vi "Print PDFCreator.vi"(0 "report in":refnum<class "NI_report.lvclass">, 2 "Printer name":string="PDFCreator", 5 "Save Directory":path, 7 "Save Filename":string="TEST", 11 "error in (no error)":errorcluster) -> (4 "report out":refnum<class "NI_report.lvclass">, 8 "File path":path, 15 "error out":errorcluster)   [LabVIEW 2010]
doc: "Jean-Marc Simard \nJanuary 6, 2010"
uses:
  <vilib>/Utility/NIReport.llb/NI_report.lvclass
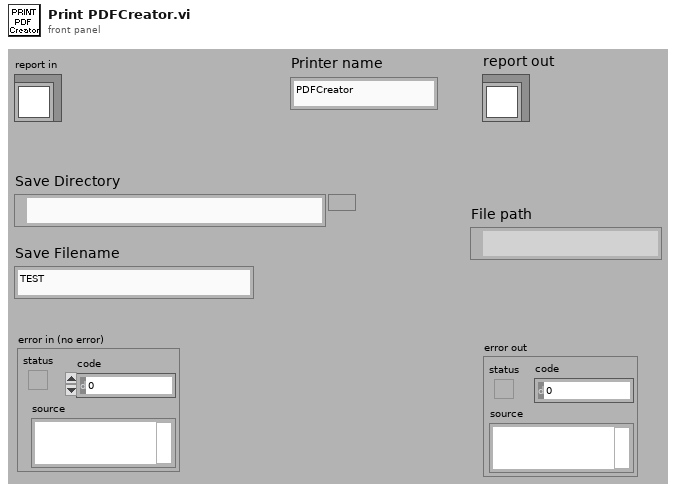
[diagram p1: front panel]
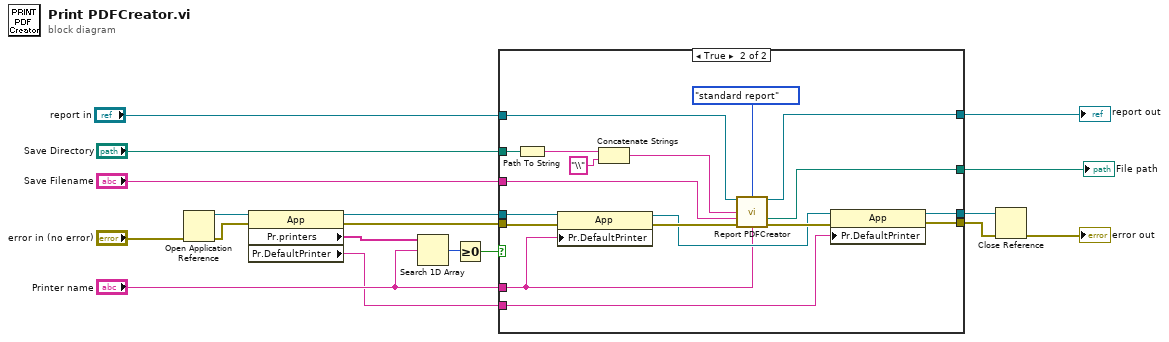
[diagram p0: block diagram]
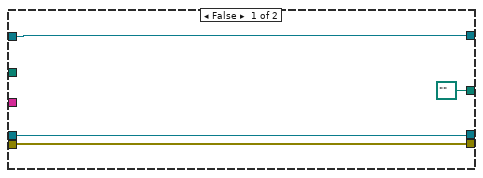
[diagram p2: hidden frame]
diagram:
  n1 = Open Application Reference(8:"error in (no error)") -> (0:w13:errorcluster, 3:w12:refnum<vi>)  [unwired: 3 out]
  n2 = property class="App"(reference=w12, error in=w13) -> (reference out=w8:refnum<vi>, error out=w7:errorcluster, "Pr.printers"=w11:string[], "Pr.DefaultPrinter"=w6:string)
  n3 = Search 1D Array(1D array=w11, element="Printer name") -> (index of element=w10:i32)  [unwired: 1 out]
  n4 = Greater Or Equal To 0?(x=w10) -> (x >= 0?=w9:bool)
  n5 = case shown="True" w9 {
    tunnel: w8 -> [w22 w40]
    tunnel: w7 -> [w21 w39]
    tunnel: "Printer name" -> [_ w23]
    tunnel: w6 -> [_ w25]
    tunnel: "Save Filename" -> [_ w35]
    tunnel: "Save Directory" -> [_ w34]
    tunnel: [w22 w33] -> w5
    tunnel: [w21 w32] -> w4
    tunnel: "report in" -> [w20 w28]
    tunnel: [w20 w27] -> w2
    tunnel: [path "" ("File path") w26] -> w1
    frame False {
    }
    frame True {
      n6 = Path To String(path=w34) -> (string=w31:string)
      n7 = property class="App"(reference=w40, error in=w39, "Pr.DefaultPrinter"=w23) -> (reference out=w36:refnum<vi>, error out=w38:errorcluster)
      n8 = Concatenate Strings(w31, "\\" ("string")) -> (w30:string)
      n9 = call "Report PDFCreator.vi"("report in"=w28, "Conversion to PDF"=enum16{"standard report", "file"}."standard report", "AutosaveDirectory"=w30, "AutosaveFilename"=w35, "error in (no error)"=w38, "Printer name"=w23) -> ("report out"=w27:refnum<class "NI_report.lvclass">, "File path"=w26:path, "error out"=w37:errorcluster)  [unwired: 7 out]
      n10 = property class="App"(reference=w36, error in=w37, "Pr.DefaultPrinter"=w25) -> (reference out=w33:refnum<vi>, error out=w32:errorcluster)
    }
  }
  "report out" <- w2
  "File path" <- w1
  n11 = Close Reference(reference=w5, error in (no error)=w4) -> (error out=→"error out":errorcluster)
